vi "MM6.ScanStep.vi"(0 "i ref in":refnum<vi>, 3 "ms timeout (10000)":i32=10000, 5 "error in (no error)":errorcluster) -> (14 "i ref out":refnum<vi>, 17 "timed out":bool, 19 "error out":errorcluster)   [LabVIEW 2014, in "MM6.lvlib"]
doc: "This is the method that makes the scan steps. The actual step is stored in the attributes."
uses:
  MM6.lvlib
  CS_Core/CSSystem/CoreDefs/CoreDefs.call_type.ctl
  CS_Core/BaseProcess/BaseProcess.descriptor string definition.ctl
  CS_Core/CSSystem/CoreDefs/CoreDefs.rawDataType.ctl
  CS_Core/BaseProcess/BaseProcess.lvlib
panel:
  in  "CallClusterTyp":T1={"Object"="", "Selector"="", "CallType"=enum."synchronous", "Async Object"="", "Async Selector"="", "Data Descriptor"="", "Data"=[], "Error #"=0, "Expire"=0}
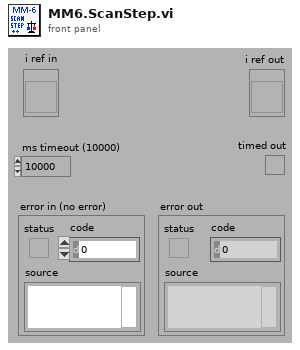
[diagram p1: front panel]
types:
  T1 = typedef "CoreDefs.call_type.ctl" = cluster{"Object":string, "Selector":string, "CallType":enum16{"simple", "synchronous", "asynchronous"}, "Async Object":string, "Async Selector":string, "Data Descriptor":T2, "Data":T3, "Error #":i32, "Expire":u32}
  T2 = typedef "BaseProcess.lvlib/BaseProcess.descriptor string definition.ctl" = string
  T3 = typedef "CoreDefs.rawDataType.ctl" = i8[]
  T4 = typedef "MM6.lvlib/MM6.i attribute.ctl" = cluster{"ConfigData":T5, "UsedObjs":string[], "ActScanStep":i32[], "AbortRequest":bool, "StopRequest":bool, "# cycles":i32, "Connected":bool, "MMStatus":T20, "# data":i32, "DIMServices":cluster{"MM6StatusString":string, "MM6StatusID":i32, "discArchiver":string, "discArchiverID":i32, "eventBuilder":string, "eventBuilderID":i32, "GUIIDString":string, "GUIIDStringID":i32}, "dataFile":string, "ExtraDataSets":T21, "PGRunning":T22}
  T5 = typedef "LEBITDefs.lvlib/LEBITDefs.ConfigData.ctl" = cluster{"GenConfig":T6, "Configs":T8[]}
  T6 = typedef "LEBITDefs.lvlib/LEBITDefs.GenConfig.ctl" = cluster{"Mode":i32, "Logs":T7[]}
  T7 = typedef "LEBITDefs.lvlib/LEBITDefs.Log.ctl" = cluster{"Name":string, "FctName":string, "Special":string}
  T8 = typedef "LEBITDefs.lvlib/LEBITDefs.OneConfig.ctl" = cluster{"MCA":T9, "Timing":T10, "Scans":T13[], "FreqDevs":T14[], "CleanDev":T15, "NrCycles":i32, "Specials":T17[], "Delays":T18[], "DAC":T19}
  T9 = typedef "LEBITDefs.lvlib/LEBITDefs.MCA.ctl" = cluster{"Name":string, "Address":string, "NrChannels":i32, "Gate":i32, "NrPipse":i32}
  T10 = typedef "LEBITDefs.lvlib/LEBITDefs.Timing.ctl" = cluster{"TimeTables":cluster{"TimeTable":T11}[], "Memories":T12[], "ScanX":string, "ScanY":string}
  T11 = typedef "LEBITDefs.lvlib/LEBITDefs.Timetable.ctl" = dbl[]
  T12 = typedef "LEBITDefs.lvlib/LEBITDefs.Memory.ctl" = cluster{"Device":string, "ExtTrig":bool, "TT2Use":i32, "PatternTable":string[]}
  T13 = typedef "LEBITDefs.lvlib/LEBITDefs.ScanDev.ctl" = cluster{"Name":string, "FctName":string, "Values":dbl[], "NrScanVals":i32, "Special":string}
  T14 = typedef "LEBITDefs.lvlib/LEBITDefs.FreqDev.ctl" = cluster{"Name":string, "Amp":dbl, "CenterFreq":dbl, "Time":dbl}
  T15 = typedef "LEBITDefs.lvlib/LEBITDefs.CleanDev.ctl" = cluster{"Name":string, "CleanData":T16[]}
  T16 = typedef "LEBITDefs.lvlib/LEBITDefs.CleanDataType.ctl" = cluster{"Amp":dbl, "Center":dbl, "Plus":dbl, "Minus":dbl, "Time":dbl}
  T17 = typedef "LEBITDefs.lvlib/LEBITDefs.Special.ctl" = cluster{"Name":string, "FctName":string, "VerySpecial":string, "Data":dbl}
  T18 = typedef "LEBITDefs.lvlib/LEBITDefs.Delay.ctl" = cluster{"Name":string, "Delay":dbl}
  T19 = typedef "LEBITDefs.lvlib/LEBITDefs.DAC.ctl" = cluster{"Name":string, "Step1":i32, "Step2":i32}
  T20 = typedef "MM6.lvlib/MM6.status.ctl" = enum16{"loaded", "load_error", "config", "config_error", "init", "init_error", "data_reset", "data_reset_error", "running", "start_error", "run_error", "abort_requested", "aborted", "stop_requested", "stopped", "stop_error", "Connected", "NOTConnected"}
  T21 = typedef "LEBITDefs.lvlib/LEBITDefs.ExtraData.ctl" = cluster{"Ions":cluster{"ExcitIonMass":string, "ExcitIonCharge":i32, "CleanIons":cluster{"CleanIonMass":string, "CleanIonCharge":i32}[]}, "TimingDescription":cluster{"TimeTableDescription":cluster{"Times":string[]}[], "PatternTableDescription":cluster{"Pattern":string[]}[]}, "ScanUnits":string[]}[]
  T22 = typedef "PPG_ABC.lvlib/PPG_ABC.PG_Running.ctl" = i32
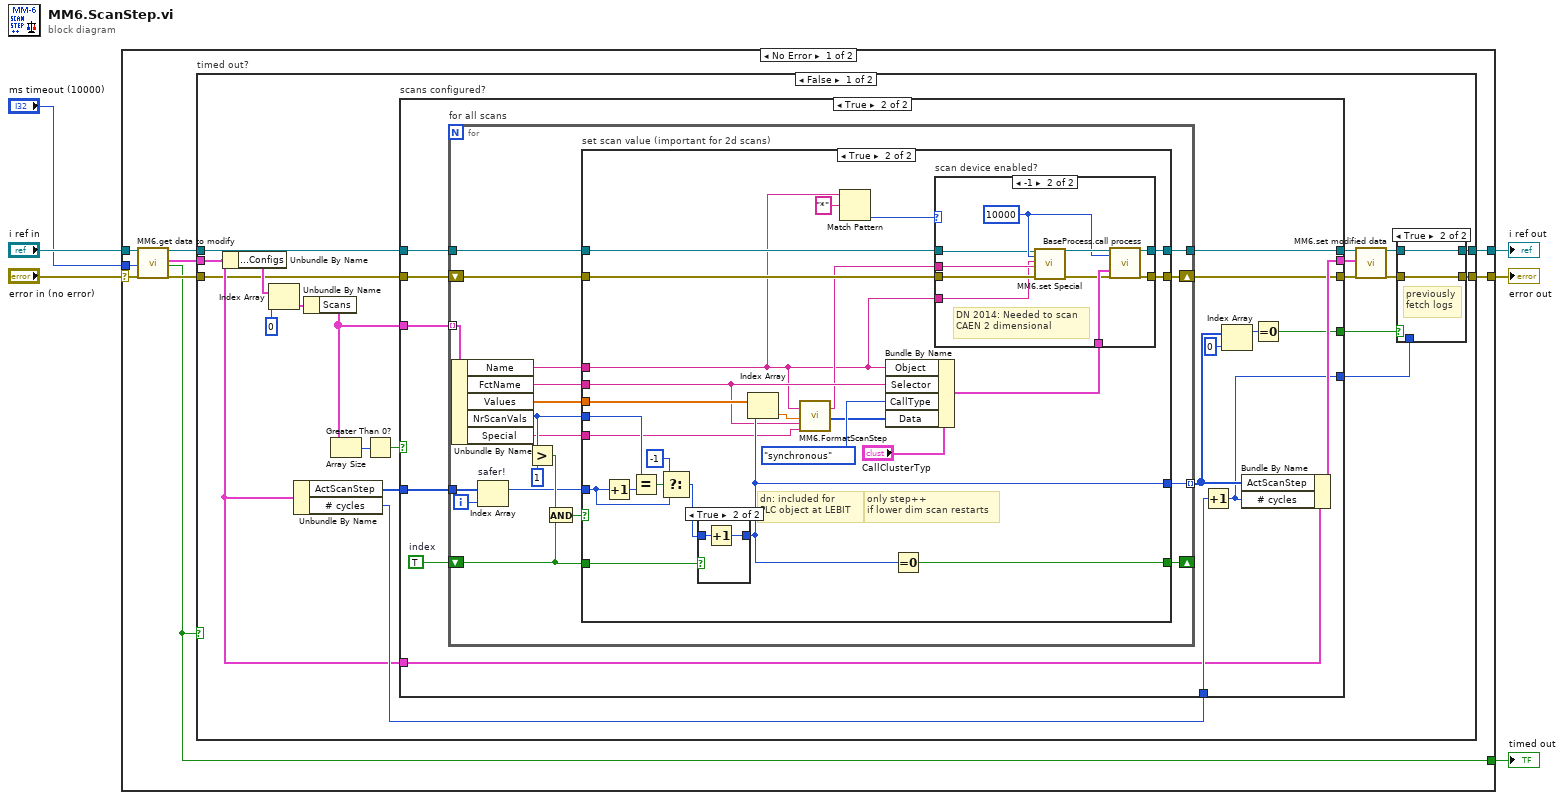
[diagram p0: block diagram]
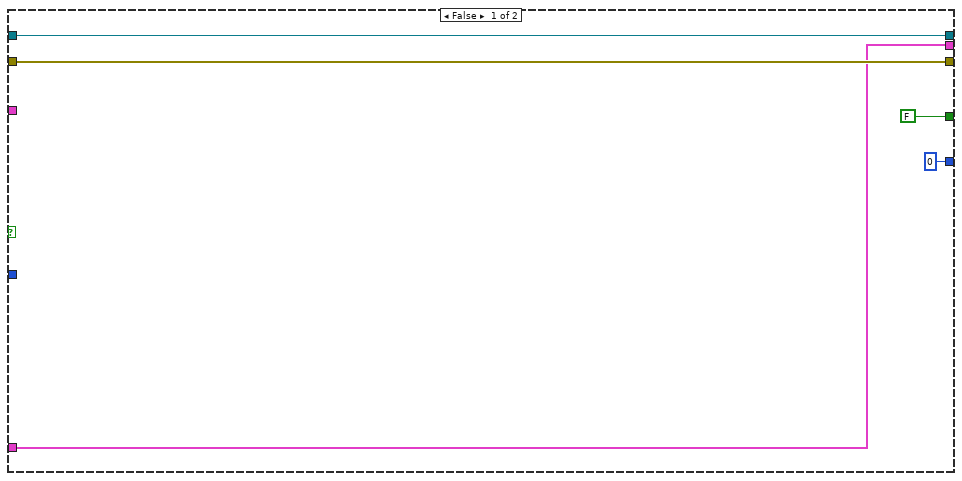
[diagram p3: hidden frame]
diagram:
  n1 = case shown="No Error" "error in (no error)" {
    selector: "error in (no error)" -> [w7 w125]
    tunnel: "i ref in" -> [w15 w126]
    tunnel: [w14 w125] -> w5
    tunnel: [w13 w126] -> w4
    tunnel: "ms timeout (10000)" -> [w9 _]
    tunnel: [w8 _] -> w2
    frame No Error {
      n2 = call "MM6.get data to modify.vi"("i ref in"=w15, "ms timeout (10000)"=w9, "error in (no error)"=w7) -> ("i ref out"=w12:refnum<vi>, "i attribute"=w10:T4, "timed out"=w8:bool, "error out"=w11:errorcluster)  [unwired: 13 in]
      n3 = case "timed out?" shown="False" w8 {
        tunnel: [w17 w123] -> w14
        tunnel: [w19 w124] -> w13
        tunnel: w12 -> [w23 w124]
        tunnel: w11 -> [w22 w123]
        tunnel: w10 -> [w28 _]
        frame False {
          n4 = Unbundle By Name(w28) -> ("ConfigData.Configs"=w26:T8[])
          n5 = Index Array(array=w26, index=0 ("NrConfig")) -> (element=w25:T8)
          n6 = Unbundle By Name(w28) -> ("ActScanStep"=w31:i32[], "# cycles"=w29:i32)
          n7 = Unbundle By Name(w25) -> ("Scans"=w24:T13[])
          n8 = Array Size(array=w24) -> (size(s)=w34:i32)
          n9 = Greater Than 0?(x=w34) -> (x > 0?=w35:bool)
          n10 = case "scans configured?" shown="True" w35 {
            tunnel: w23 -> [w44 w59]
            tunnel: [w44 w58] -> w33
            tunnel: w22 -> [w43 w52]
            tunnel: [w43 w51] -> w32
            tunnel: w24 -> [_ w57]
            tunnel: w31 -> [_ w56]
            tunnel: w28 -> [w42 w45]
            tunnel: [w42 w55] -> w30
            tunnel: w29 -> [_ w53]
            tunnel: [FALSE w47] -> w21
            tunnel: [0 w46] -> w16
            frame False {
            }
            frame True {
              w54 = TRUE  # index
              n11 = for "for all scans" {
                tunnel: w59 -> [w78]
                tunnel: [w77] -> w58
                tunnel: w57 -> [w76] mode=indexing
                tunnel: w56 -> [w73]
                tunnel: [w72] -> w50 mode=indexing
                shift-right: [w71] -> _
                shift-left: w54 -> [w65]
                shift-right: [w61] -> w51
                shift-left: w52 -> [w62]
                i -> [w63]
                n12 = Unbundle By Name(w76) -> ("Name"=w70:string, "FctName"=w75:string, "Values"=w74:dbl[], "NrScanVals"=w69:i32, "Special"=w60:string)
                n13 = Index Array "safer!"(array=w73, index=w63) -> (element=w64:i32)
                n14 = Greater?(x=w69, y=1) -> (0:w67:bool)
                n15 = And(x=w67, y=w65) -> (x .and. y?=w66:bool)
                n16 = case "set scan value (important for 2d scans)" shown="True" w66 {
                  tunnel: w78 -> [w82 w107]
                  tunnel: [w82 w106] -> w77
                  tunnel: w62 -> [w81 w105]
                  tunnel: [w81 w104] -> w61
                  tunnel: w75 -> [_ w86]
                  tunnel: w74 -> [_ w102]
                  tunnel: w64 -> [w80 w93]
                  tunnel: w70 -> [_ w83]
                  tunnel: [w80 w90] -> w72
                  tunnel: [w79 w89] -> w71
                  tunnel: w65 -> [w79 w98]
                  tunnel: w69 -> [_ w92]
                  tunnel: w60 -> [_ w85]
                  frame False {
                  }
                  frame True {
                    # "dn: included for\nPLC object at LEBIT"
                    # "only step++\nif lower dim scan restarts"
                    n17 = Increment(x=w93) -> (x+1=w94:i32)
                    n18 = Equal?(x=w92, y=w94) -> (x = y?=w91:bool)
                    n19 = Select(t=-1, s=w91, f=w93) -> (s? t:f=w95:i32)
                    n20 = case shown="True" w98 {
                      tunnel: w95 -> [w120 w122]
                      tunnel: [w120 w121] -> w90
                      frame False {
                      }
                      frame True {
                        n21 = Increment(x=w122) -> (x+1=w121:i32)
                      }
                    }
                    n22 = Index Array(array=w102, index=w90) -> (element=w88:dbl)
                    n23 = call "MM6.FormatScanStep.vi"("Name"=w83, "Value"=w88, "FctName"=w86, "SetSpecial"=w85) -> ("SetSpecial"=w84:string, "byteArray out"=w87:T3)  [unwired: 14 in]
                    n24 = Match Pattern(string=w83, regular expression="*") -> (offset past match=w96:i32)  [unwired: 1 in, 3 out]
                    n25 = Bundle By Name(cluster="CallClusterTyp", "Object"=w83, "Selector"=w86, "CallType"=enum16{"simple", "synchronous", "asynchronous"}."synchronous", "Data"=w87) -> (w100:T1)
                    n26 = Equal To 0?(x=w90) -> (x = 0?=w89:bool)
                    n27 = case "scan device enabled?" shown="-1" w96 {
                      tunnel: w107 -> [w109 w112]
                      tunnel: [w109 w119] -> w106
                      tunnel: w105 -> [w108 w116]
                      tunnel: [w108 w118] -> w104
                      tunnel: w100 -> [_ w117]
                      tunnel: w84 -> [_ w111]
                      tunnel: w83 -> [_ w110]
                      frame 0, Default {
                      }
                      frame -1 {
                        w113 = 10000 ("timeout (ms)")
                        # "DN 2014: Needed to scan\nCAEN 2 dimensional"
                        n28 = call "MM6.set Special.vi"("i ref in"=w112, "ms timeout (10000)"=w113, "Object"=w110, "Special"=w111, "error in (no error)"=w116) -> ("i ref out"=w114:refnum<vi>, "error out"=w115:errorcluster)  [unwired: 12 in, 1 out]
                        n29 = call "BaseProcess.call process.vi"("i ref in"=w114, "timeout (ms)"=w113, "call cluster in"=w117, "error in (no error)"=w115) -> ("i ref out"=w119:refnum<vi>, "error out"=w118:errorcluster)  [unwired: 13 in, 1 out]
                      }
                    }
                  }
                }
              }
              n30 = Increment(x=w53) -> (x+1=w46:i32)
              n31 = Index Array ("safer!")(array=w50, index=0) -> (element=w48:i32)
              n32 = Bundle By Name(cluster=w45, "ActScanStep"=w50, "# cycles"=w46) -> (w55:T4)
              n33 = Equal To 0?(x=w48) -> (x = 0?=w47:bool)
            }
          }
          n34 = call "MM6.set modified data.vi"("i ref in"=w33, "i attribute"=w30, "error in (no error)"=w32) -> ("i ref out"=w20:refnum<vi>, "error out"=w18:errorcluster)  [unwired: 15 in]
          n35 = case shown="True" w21 {
            tunnel: w20 -> [w37 w39]
            tunnel: [w37 w39] -> w19
            tunnel: w18 -> [w36 w38]
            tunnel: [w36 w38] -> w17
            tunnel: w16 -> [_ _]
            frame False {
            }
            frame True {
              # "previously\nfetch logs"
            }
          }
        }
        frame True {
        }
      }
    }
    frame Error {
    }
  }
  "error out" <- w5
  "i ref out" <- w4
  "timed out" <- w2
